vi "solar_addon VISA.vi"() -> ()   [LabVIEW 2018]
doc: "This addon queries a VISA session."
uses:
  solar/solar_ctl SOLAR Refnum.ctl
panel:
  in  "Command List":u16(ring) items=["Select Query...", "*IDN?", "*CLS", "*RST", "*STB?"]
  in  "VISA Timeout":u32 format="%d ms"
  in  "Read Wait":u32 format="%d ms"
  out "Bytes Recieved":u32
  in  "Bytes Expected":u32
  out "Received Time":string
  out "Status":string
  in  "Clear":bool
  in  "Write":string
  out "Read":string
  out "Error":errorcluster
  in  "Query":bool
  in  "VISA":refnum<visa-resource-name>
  in  "Variant":variant
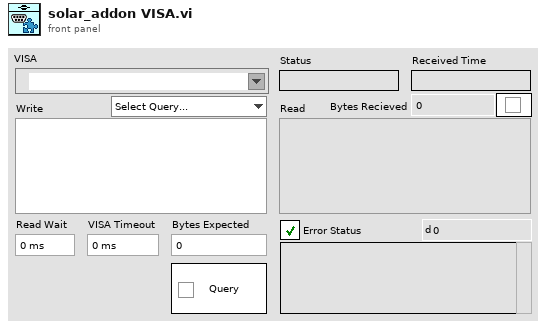
[diagram p1: front panel]
types:
  T1 = typedef "solar_ctl SOLAR Refnum.ctl" = refnum<k1>
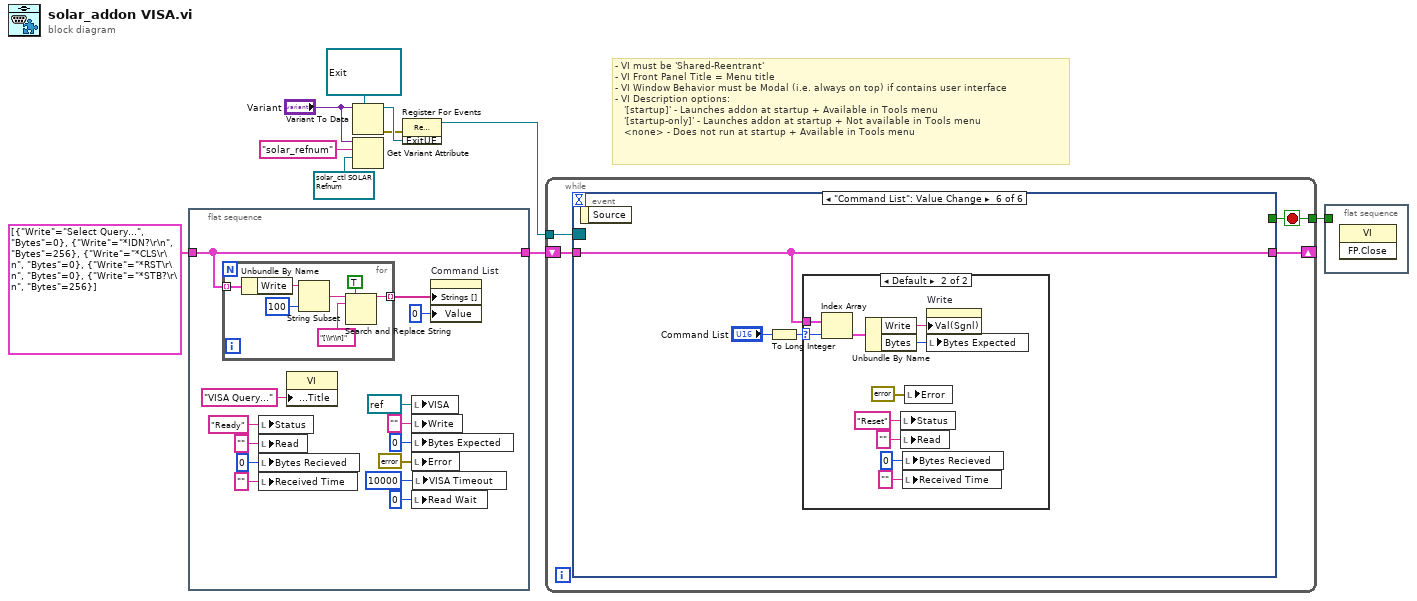
[diagram p0: block diagram]
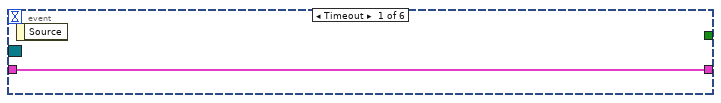
[diagram p2: hidden frame]
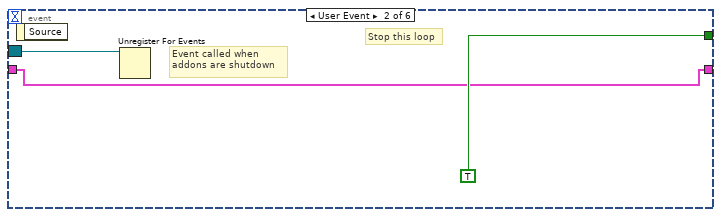
[diagram p3: hidden frame]
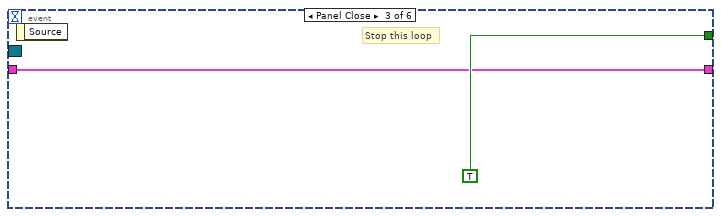
[diagram p4: hidden frame]
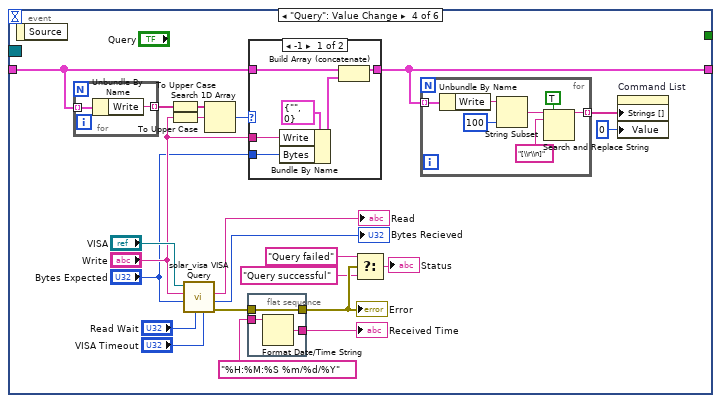
[diagram p5: hidden frame]
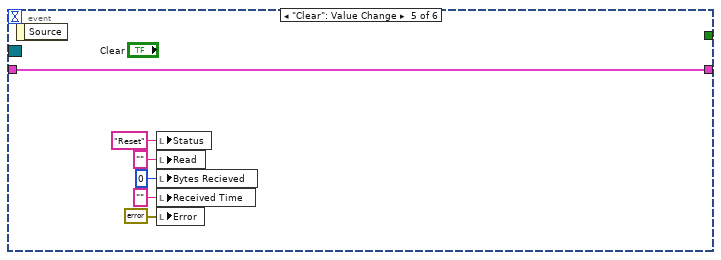
[diagram p7: hidden frame]
diagram:
  w2 = T1 refnum items=["solar"] ("SOLAR Refnum")
  # "- VI must be 'Shared-Reentrant'\n- VI Front Panel Title = Menu title\n- VI Window Behavior must be Modal (i.e. always on top) if contains user interface\n- VI Description options:\n   '[startup]' - Launches addon at startup + Available in Tools menu\n   '[startup-only]' - Launches addon at startup + Not available in Tools menu\n   <none> - Does not run at startup + Available in Tools menu"
  n1 = flat-sequence {
    tunnel: [w13] -> w5
    tunnel: cluster{"Write":string, "Bytes":u32}[] [{"Write"="Select Query...", "Bytes"=0}, {"Write"="*IDN?\r\n", "Bytes"=256}, {"Write"="*CLS\r\n", "Bytes"=0}, {"Write"="*RST\r\n", "Bytes"=0}, {"Write"="*STB?\r\n", "Bytes"=256}] -> [w13]
    frame #0 {
      n2 = for {
        tunnel: w13 -> [w31] mode=indexing
        tunnel: [w25] -> w12 mode=indexing
        n3 = Unbundle By Name(w31) -> ("Write"=w26:string)
        n4 = String Subset(string=w26, length (rest)=100 ("length (rest)")) -> (substring=w27:string)  [unwired: 1 in]
        n5 = Search and Replace String(replace all?=TRUE, input string=w27, search string="[\\r\\n]") -> (result string=w25:string)  [unwired: 5 in, 3 out]
      }
      n6 = local write "Status"("Ready" ("Status")) -> ()
      n7 = local write "Read"("" ("Read")) -> ()
      n8 = local write "Bytes Recieved"(u32 0 ("Bytes Recieved")) -> ()
      n9 = local write "Received Time"("" ("Received Time")) -> ()
      n10 = property class="VI"("Front Panel.Title"="VISA Query..." ("Front Panel Window:Title")) -> ()  [unwired: 2 in, 2 out]
      n11 = local write "VISA"(refnum<visa-resource-name> refnum ("VISA")) -> ()
      n12 = local write "Write"("" ("Write")) -> ()
      n13 = local write "Bytes Expected"(u32 0 ("Bytes Expected")) -> ()
      n14 = local write "Error"(errorcluster {"status"=FALSE, "code"=0, "source"=""} ("Error")) -> ()
      n15 = local write "Read Wait"(u32 0 ("Read Wait")) -> ()
      n16 = local write "VISA Timeout"(u32 10000 ("VISA Timeout")) -> ()
      n17 = property on="Command List" class="Ring (strict)"("Strings []"=w12, "Value"=u16 0) -> ()  [unwired: 2 in, 2 out]
    }
  }
  n18 = Variant To Data(type=refnum<user-event> refnum ("ExitUE"), Variant="Variant") -> (data=w8:refnum<user-event>, error out=w7:errorcluster)  [unwired: 1 in]
  n19 = Get Variant Attribute(Variant="Variant", name="solar_refnum", default value (empty Variant)=w2) -> ()  [unwired: 1 in, 4 out]
  n20 = register-events(error in=w7, w8) -> (reference out=w10:refnum<event-registration>)  [unwired: 1 in, 1 out]
  n21 = while {
    tunnel: w10 -> [w35]
    tunnel: [w34] -> w6
    shift-right: [w33] -> _
    shift-left: w5 -> [w32]
    stop <- w34 stop-if-true
    n22 = event shown="[5] \"Command List\": Value Change" {
      selector: w35 -> [_ w39 _ _ _ _]
      dyn-events: _ -> [_ _ _ _ _ _]
      timeout: _ -> [_ _ _ _ _ _]
      tunnel: [_ TRUE TRUE _ _ _] -> w34
      tunnel: [w36 w37 w40 w45 w83 w90] -> w33
      tunnel: w32 -> [w36 w37 w40 w44 w83 w90]
      event Timeout {
        n23 = event-data() -> ()  [unwired: 1 in, 1 out]
      }
      event User Event {
        # "Stop this loop"
        # "Event called when\naddons are shutdown"
        n24 = event-data() -> ()  [unwired: 1 in, 1 out]
        n25 = Unregister For Events(event registration refnum=w39) -> ()  [unwired: 1 in, 1 out]
      }
      event Panel Close {
        # "Stop this loop"
        n26 = event-data() -> ()  [unwired: 1 in, 1 out]
      }
      event "Query": Value Change {
        n27 = event-data() -> ()  [unwired: 1 in, 1 out]
        n28 = for {
          tunnel: w44 -> [w72] mode=indexing
          tunnel: [w71] -> w49 mode=indexing
          n29 = Unbundle By Name(w72) -> ("Write"=w71:string)
        }
        n30 = To Upper Case(1:w49) -> (0:w48:string[])
        n31 = To Upper Case(1:"Write") -> (0:w47:string)
        n32 = call "solar_visa VISA Query.vi"("VISA Read Timeout (0 = Ignore)"="VISA Timeout", "ms Read Wait (0)"="Read Wait", "Bytes Expected (0 = No Read)"="Bytes Expected", "Write (\"\" = No Write)"="Write", "VISA Resource in"="VISA") -> ("error out"=w60:errorcluster, "Bytes Recieved"=→"Bytes Recieved":u32, "Read"=→"Read":string)  [unwired: 3 in, 1 out]
        n33 = Search 1D Array(1D array=w48, element=w47) -> (index of element=w46:i32)  [unwired: 1 in]
        n34 = flat-sequence {
          tunnel: [w82] -> w55
          tunnel: w60 -> [w82]
          tunnel: [w81] -> w58
          tunnel: "%H:%M:%S %m/%d/%Y" ("time format string (%c)") -> [w80]
          frame #0 {
            n35 = Format Date/Time String(time format string (%c)=w80) -> (date/time string=w81:string)  [unwired: 2 in]
          }
        }
        n36 = case shown="-1" w46 {
          tunnel: [w68 w70] -> w45
          tunnel: w44 -> [w69 w70]
          tunnel: "Write" -> [w65 _]
          tunnel: "Bytes Expected" -> [w64 _]
          frame -1 {
            n37 = Bundle By Name(cluster=cluster{"Write":string, "Bytes":u32} {"Write"="", "Bytes"=0} ("Query 2"), "Write"=w65, "Bytes"=w64) -> (w66:cluster{"Write":string, "Bytes":u32})
            n38 = Build Array (concatenate)(w69, w66) -> (w68:cluster{"Write":string, "Bytes":u32}[])
          }
          frame Default {
          }
        }
        n39 = Select(t="Query failed", s=w55, f="Query successful") -> (s? t:f=→"Status":string)
        n40 = for {
          tunnel: w45 -> [w79] mode=indexing
          tunnel: [w73] -> w50 mode=indexing
          n41 = Unbundle By Name(w79) -> ("Write"=w74:string)
          n42 = String Subset(string=w74, length (rest)=100 ("length (rest)")) -> (substring=w75:string)  [unwired: 1 in]
          n43 = Search and Replace String(replace all?=TRUE, input string=w75, search string="[\\r\\n]") -> (result string=w73:string)  [unwired: 5 in, 3 out]
        }
        n44 = property on="Command List" class="Ring (strict)"("Strings []"=w50, "Value"=u16 0) -> ()  [unwired: 2 in, 2 out]
        "Error" <- w55
        "Received Time" <- w58
      }
      event "Clear": Value Change {
        n45 = event-data() -> ()  [unwired: 1 in, 1 out]
        n46 = local write "Status"("Reset" ("Status")) -> ()
        n47 = local write "Read"("" ("Read")) -> ()
        n48 = local write "Bytes Recieved"(u32 0 ("Bytes Recieved")) -> ()
        n49 = local write "Received Time"("" ("Received Time")) -> ()
        n50 = local write "Error"(errorcluster {"status"=FALSE, "code"=0, "source"=""} ("Error")) -> ()
      }
      event "Command List": Value Change {
        n51 = event-data() -> ()  [unwired: 1 in, 1 out]
        n52 = To Long Integer(number="Command List") -> (32bit integer=w89:i32)
        n53 = case shown="Default" w89 {
          selector: w89 -> [_ w100]
          tunnel: w90 -> [_ w101]
          frame 0 {
          }
          frame Default {
            n54 = Index Array(array=w101, index=w100) -> (element=w99:cluster{"Write":string, "Bytes":u32})
            n55 = Unbundle By Name(w99) -> ("Write"=w98:string, "Bytes"=w97:u32)
            n56 = local write "Status"("Reset" ("Status")) -> ()
            n57 = local write "Read"("" ("Read")) -> ()
            n58 = local write "Bytes Recieved"(u32 0 ("Bytes Recieved")) -> ()
            n59 = local write "Received Time"("" ("Received Time")) -> ()
            n60 = local write "Error"(errorcluster {"status"=FALSE, "code"=0, "source"=""} ("Error")) -> ()
            n61 = property on="Write" class="Str"("Val(Sgnl)"=w98) -> ()  [unwired: 2 in, 2 out]
            n62 = local write "Bytes Expected"(w97) -> ()
          }
        }
      }
    }
  }
  n63 = flat-sequence {
    tunnel: w6 -> [_]
    frame #0 {
      n64 = invoke class="VI" method="FP.Close"() -> ()  [unwired: 3 in, 3 out]
    }
  }
